vi "Check for Fresh Message.vi"(8 "error in":errorcluster, 11 "Handle Laser Enable Request in":refnum<class "Handle Laser Enable Request.lvclass">) -> (0 "error out":errorcluster, 1 "Enqueuer":refnum<class "Message Enqueuer.lvclass">, 2 "Enqueuer not Valid":bool, 3 "Handle Laser Enable Request Out":refnum<class "Handle Laser Enable Request.lvclass">)   [LabVIEW 2014, in "Handle Laser Enable Request.lvclass"]
doc: "This method is a dynamic method that \n1) checks for a good connection to the shared variable. If it is not present, then it attempts to connect If a connection is not available, then this VI will do nothing.\n2) Check the state of the enqueuer. If the state is no good, return with this indication and do nothing.\n2) If the connection is good, check to see if the current shared variable state has changed.\n3) If the state has changed, pump the message into the appropriate enqueuer."
uses:
  Handle Laser Enable Request.lvclass
  <vilib>/ActorFramework/Message Enqueuer/Message Enqueuer.lvclass
  Instr Actor/Messages/Set Las Enable MSG/Set Las Enable MSG.lvclass
  Instr Actor/Messages/Set Las Enable MSG/Set Las Enable MSG.lvclass/Set Las Enable MSG.ctl
  <vilib>/ActorFramework/Message Enqueuer/Message Enqueuer.lvclass/Message Enqueuer.ctl
  Instr Actor/Messages/Set Las Enable MSG/Write Laser Enable.vi
  <vilib>/ActorFramework/Message Priority Queue/Priority Enqueue.vi
  Network Command Processor.lvclass
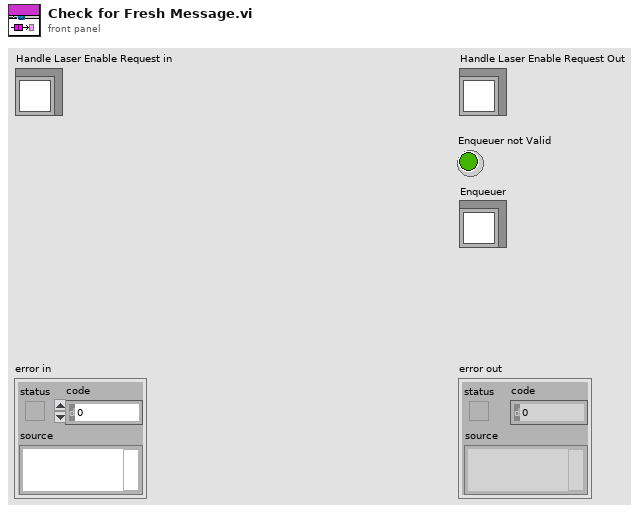
[diagram p1: front panel]
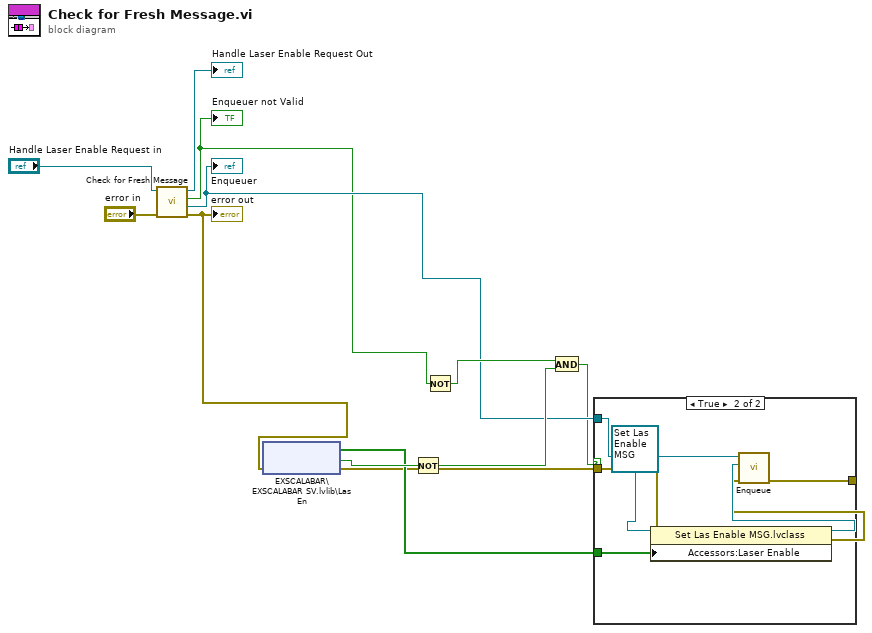
[diagram p0: block diagram]
diagram:
  n1 = call-parent "Check for Fresh Message.vi"("error in"="error in", "Network Command Processor in"="Handle Laser Enable Request in") -> ("error out"=w3:errorcluster, "Enqueuer"=w4:refnum<class "Message Enqueuer.lvclass">, "Enqueuer not Valid"=w2:bool, "Network Command Processor out"=→"Handle Laser Enable Request Out":refnum<class "Handle Laser Enable Request.lvclass">)  [unwired: 6 in]
  "error out" <- w3
  "Enqueuer not Valid" <- w2
  "Enqueuer" <- w4
  n2 = shared-variable "EXSCALABAR\\EXSCALABAR SV.lvlib\\Las En"(error in=w3) -> (w6:bool[], error out=w5:errorcluster, w9:bool)  [unwired: 1 in]
  n3 = Not(x=w9) -> (.not. x?=w7:bool)
  n4 = Not(x=w2) -> (.not. x?=w8:bool)
  n5 = And(x=w8, y=w7) -> (x .and. y?=w1:bool)
  n6 = case shown="True" w1 {
    tunnel: w4 -> [_ w18]
    tunnel: w6 -> [_ w20]
    tunnel: w5 -> [w13 w17]
    tunnel: [w13 w15] -> _
    frame False {
    }
    frame True {
      n7 = property class="Set Las Enable MSG.lvclass"(reference=refnum<class "Set Las Enable MSG.lvclass"> refnum ("Instrument Lib:Set Las Enable MSG.lvclass"), error in=w17, "Accessors:Laser Enable"=w20) -> (reference out=w19:refnum<class "Set Las Enable MSG.lvclass">, error out=w16:errorcluster)
      n8 = call <vilib>:"Enqueue.vi"("error in (no error)"=w16, "Message"=w19, "Message Enqueuer in"=w18) -> ("error out"=w15:errorcluster)  [unwired: 7 in, 1 out]
    }
  }
